vi "OAT Index 2D XY Signal.vi"(0 "2D XY signal":cluster{"X":dbl[], "Y":dbl[]}[][](array[cluster]) {"Y" format="%.2f"; "X" format="%.2f"}, 1 "index selection":u16(ring) items=["Index Channel", "Index Order"], 5 "channel or order index (0)":i32, 11 "error in (no error)":errorcluster) -> (4 "XY signal out":cluster{"X":dbl[], "Y":dbl[]}[](array[cluster]) {"Y" format="%.2f"; "X" format="%.2f"}, 15 "error out":errorcluster)   [LabVIEW 2017, in "SoundVib_OAUtility.lvlib"]
doc: "Returns a 1D XY signal array of a 2D XY signal array at a specific channel or order. This VI uses the row or column index value to determine which signal array to return."
uses:
  <vilib>/addons/Sound and Vibration/Order Analysis/Utility/SoundVib_OAUtility.lvlib
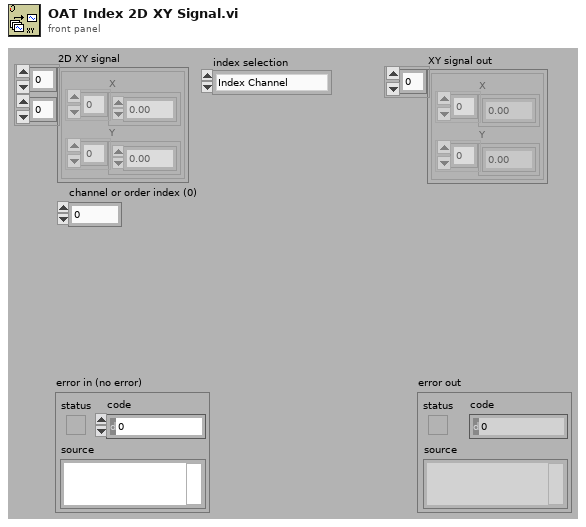
[diagram p1: front panel]
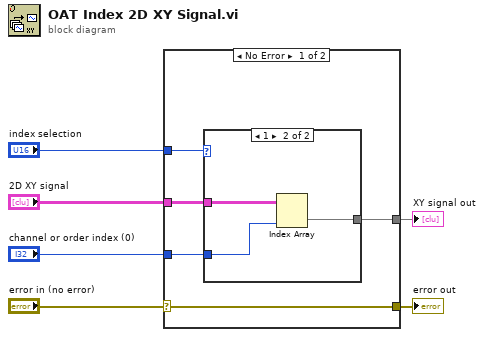
[diagram p0: block diagram]
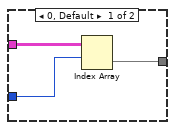
[diagram p2: hidden frame]
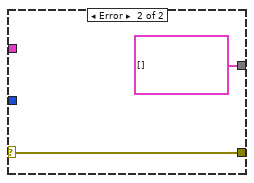
[diagram p3: hidden frame]
diagram:
  n1 = case shown="No Error" "error in (no error)" {
    selector: "error in (no error)" -> [w11 w19]
    tunnel: [w11 w19] -> w5
    tunnel: "index selection" -> [w10 _]
    tunnel: "2D XY signal" -> [w9 _]
    tunnel: "channel or order index (0)" -> [w8 _]
    tunnel: [w7 cluster{"X":dbl[], "Y":dbl[]}[] [] ("2D XY signal")] -> w1
    frame No Error {
      n2 = case shown="1" w10 {
        tunnel: w9 -> [w14 w17]
        tunnel: w8 -> [w13 w16]
        tunnel: [w12 w15] -> w7
        frame 0, Default {
          n3 = Index Array(array=w14, index (row)=w13) -> (element=w12:cluster{"X":dbl[], "Y":dbl[]}[])  [unwired: 1 in]
        }
        frame 1 {
          n4 = Index Array(array=w17, index (col)=w16) -> (element=w15:cluster{"X":dbl[], "Y":dbl[]}[])  [unwired: 1 in]
        }
      }
    }
    frame Error {
    }
  }
  "error out" <- w5
  "XY signal out" <- w1
